vi "Check_Server.vi"(3 "timeout ms (60000)":i32, 5 "address":string) -> (1 "OK":bool)   [LabVIEW 2011]
panel:
  out "error out":errorcluster
  out "connection ID":refnum<k5>
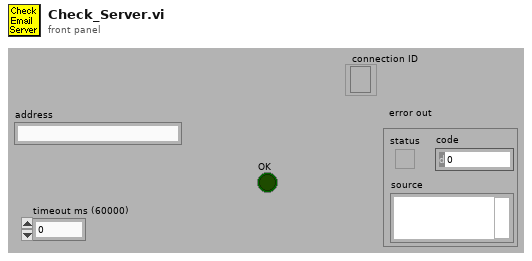
[diagram p1: front panel]
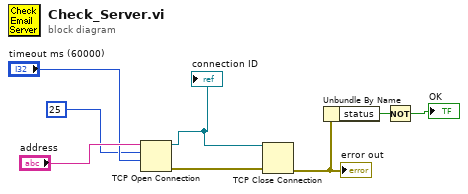
[diagram p0: block diagram]
diagram:
  n1 = TCP Open Connection(address="address", remote port or service name=u16 25 ("remote port"), timeout ms (60000)="timeout ms (60000)") -> (connection ID=w6:refnum<k5>, error out=w5:errorcluster)  [unwired: 1 in, 1 out]
  "connection ID" <- w6
  n2 = TCP Close Connection(connection ID=w6, error in (no error)=w5) -> (error out=w4:errorcluster)  [unwired: 2 out]
  "error out" <- w4
  n3 = Unbundle By Name(w4) -> ("status"=w3:bool)
  n4 = Not(x=w3) -> (.not. x?=→"OK":bool)
